vi "Drum Subvi.vi"(0 "Yellow Line":T2={"Global Rectangle"=[342, 292, 349, 377], "Contours"=[{"ID"=enum."External", "Type"=2, "Coordinates"=[342, 376, 348, 292]}]} {"Contours"."Type" items=["No Selection", "Point", "Line", "Rectangle", "Oval", "Polygon", "Freehand Region", "Annulus", "Unused2", "Unused3", "Broken Line", "Freehand Line", "Rotated Rectangle"]}, 1 "Green Line":T2={"Global Rectangle"=[406, 309, 423, 383], "Contours"=[{"ID"=enum."External", "Type"=2, "Coordinates"=[422, 382, 406, 309]}]} {"Contours"."Type" items=["No Selection", "Point", "Line", "Rectangle", "Oval", "Polygon", "Freehand Region", "Annulus", "Unused2", "Unused3", "Broken Line", "Freehand Line", "Rotated Rectangle"]}, 3 "Red Line":T2={"Global Rectangle"=[300, 297, 320, 380], "Contours"=[{"ID"=enum."External", "Type"=2, "Coordinates"=[300, 379, 319, 297]}]} {"Contours"."Type" items=["No Selection", "Point", "Line", "Rectangle", "Oval", "Polygon", "Freehand Region", "Annulus", "Unused2", "Unused3", "Broken Line", "Freehand Line", "Rotated Rectangle"]}, 8 "Image Dst Out":T1, 12 "Blue Line":T2={"Global Rectangle"=[374, 278, 383, 377], "Contours"=[{"ID"=enum."External", "Type"=2, "Coordinates"=[382, 376, 374, 278]}]} {"Contours"."Type" items=["No Selection", "Point", "Line", "Rectangle", "Oval", "Polygon", "Freehand Region", "Annulus", "Unused2", "Unused3", "Broken Line", "Freehand Line", "Rotated Rectangle"]}, 14 "error out":errorcluster) -> (7 "LED Red":bool, 9 "Yellow Array":bool[](array[boolean]), 13 "Foot Pedal":bool, 16 "Blue array":bool[](array[boolean]), 17 "Red Array":bool[](array[boolean]), 20 "Green Array":bool[](array[boolean]), 23 "Blue Drum 2":bool, 24 "Yellow Drum":bool, 25 "Green Drum":bool, 27 "error out 2":errorcluster)   [LabVIEW 2009]
uses:
  <vilib>/vision/Image Controls.llb/IMAQ Image.ctl
  <vilib>/Analysis/3filter.llb/Filter Passband Type.ctl
  <vilib>/Analysis/3filter.llb/Butterworth Filter (DBL).vi
  <vilib>/Analysis/NI_AALBase.lvlib
  <vilib>/vision/NI_Vision_Development_Module.lvlib
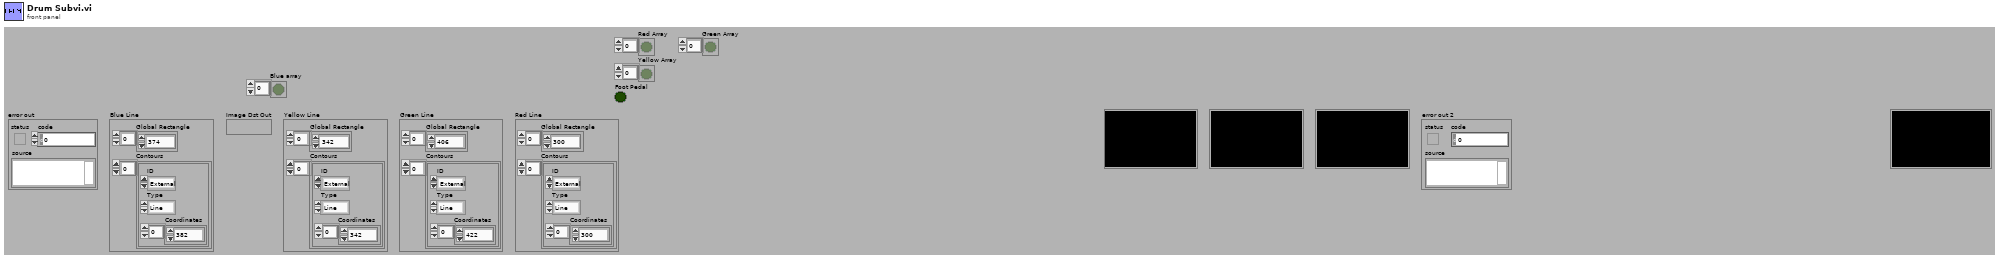
[diagram p1: front panel]
types:
  T1 = typedef "IMAQ Image.ctl" = refnum<image>
  T2 = cluster{"Global Rectangle":i32[], "Contours":cluster{"ID":enum32{"External", "Internal"}, "Type":u32, "Coordinates":i32[]}[]}
  T3 = typedef "NI_AALBase.lvlib/Filter Passband Type.ctl" = enum32{"Lowpass", "Highpass", "Bandpass", "Bandstop"}
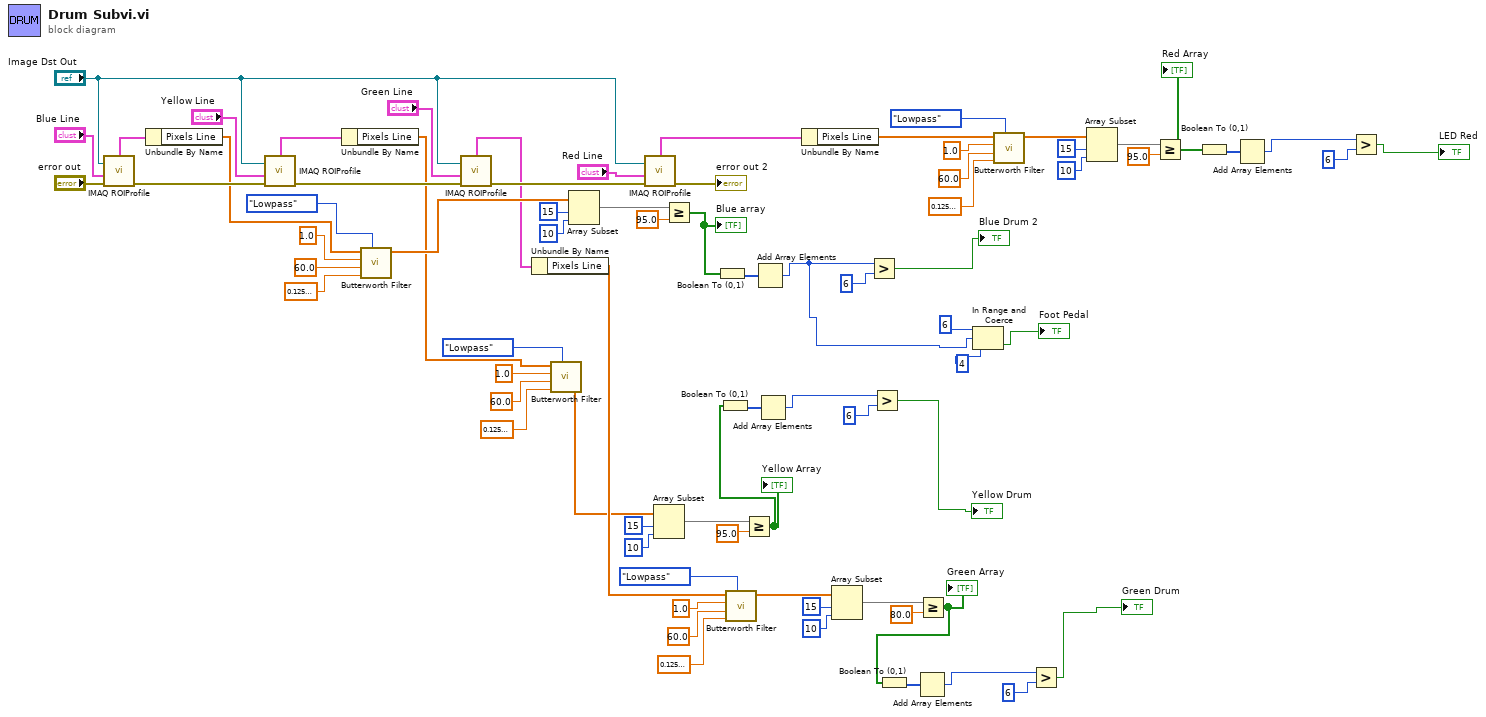
[diagram p0: block diagram]
diagram:
  n1 = call "IMAQ ROIProfile"("error in (no error)"="error out", "ROI Descriptor"="Blue Line", "Image"="Image Dst Out") -> ("error out"=w45:errorcluster, "ROI Graph"=w46:cluster{"x0":sgl, "dx":sgl, "Pixels Line":sgl[]})  [unwired: 4 out]
  n2 = Unbundle By Name(w46) -> ("Pixels Line"=w27:sgl[])
  n3 = call "IMAQ ROIProfile"("error in (no error)"=w45, "ROI Descriptor"="Yellow Line", "Image"="Image Dst Out") -> ("error out"=w74:errorcluster, "ROI Graph"=w42:cluster{"x0":sgl, "dx":sgl, "Pixels Line":sgl[]})  [unwired: 4 out]
  n4 = Unbundle By Name(w42) -> ("Pixels Line"=w39:sgl[])
  n5 = call-poly <vilib>:"Butterworth Filter.vi"("filter type"=Filter_Passband_Type."Lowpass", "low cutoff freq: fl"=0.12500000000000006 ("low"), "high cutoff freq: fh"=60.0 ("high"), "sampling freq: fs"=1.0 ("sampling"), "X"=w27) -> ("Filtered X"=w58:dbl[])  [unwired: 3 in, 1 out]
  n6 = call "IMAQ ROIProfile"("error in (no error)"=w74, "ROI Descriptor"="Green Line", "Image"="Image Dst Out") -> ("error out"=w71:errorcluster, "ROI Graph"=w48:cluster{"x0":sgl, "dx":sgl, "Pixels Line":sgl[]})  [unwired: 4 out]
  n7 = Unbundle By Name(w48) -> ("Pixels Line"=w51:sgl[])
  n8 = call-poly <vilib>:"Butterworth Filter.vi"("filter type"=Filter_Passband_Type."Lowpass", "low cutoff freq: fl"=0.12500000000000006 ("low  2"), "high cutoff freq: fh"=60.0 ("high 2"), "sampling freq: fs"=1.0 ("sampling 2"), "X"=w39) -> ("Filtered X"=w43:dbl[])  [unwired: 3 in, 1 out]
  n9 = Array Subset(array=w58, index=15, length=10) -> (w33:dbl[])
  n10 = call "IMAQ ROIProfile"("error in (no error)"=w71, "ROI Descriptor"="Red Line", "Image"="Image Dst Out") -> ("error out"=→"error out 2":errorcluster, "ROI Graph"=w69:cluster{"x0":sgl, "dx":sgl, "Pixels Line":sgl[]})  [unwired: 4 out]
  n11 = Array Subset(array=w43, index=15, length=10) -> (w36:dbl[])
  n12 = Greater Or Equal?(x=w33, y=95.0) -> (x >= y?=w21:bool[])
  "Blue array" <- w21
  n13 = Boolean To (0,1)(Boolean=w21) -> (0, 1=w20:i16[])
  n14 = call-poly <vilib>:"Butterworth Filter.vi"("filter type"=Filter_Passband_Type."Lowpass", "low cutoff freq: fl"=0.12500000000000006 ("low  3"), "high cutoff freq: fh"=60.0 ("high 3"), "sampling freq: fs"=1.0 ("sampling 3"), "X"=w51) -> ("Filtered X"=w47:dbl[])  [unwired: 3 in, 1 out]
  n15 = Greater Or Equal?(x=w36, y=95.0) -> (x >= y?=w7:bool[])
  "Yellow Array" <- w7
  n16 = Boolean To (0,1)(Boolean=w7) -> (0, 1=w14:i16[])
  n17 = Add Array Elements(numeric array=w20) -> (sum=w4:i16)
  n18 = Add Array Elements(numeric array=w14) -> (sum=w13:i16)
  n19 = Unbundle By Name(w69) -> ("Pixels Line"=w66:sgl[])
  n20 = Array Subset(array=w47, index=15, length=10) -> (w54:dbl[])
  n21 = Greater?(x=w4, y=6) -> (0:→"Blue Drum 2":bool)
  n22 = Greater?(x=w13, y=6) -> (0:→"Yellow Drum":bool)
  n23 = Greater Or Equal?(x=w54, y=80.0) -> (x >= y?=w8:bool[])
  "Green Array" <- w8
  n24 = Boolean To (0,1)(Boolean=w8) -> (0, 1=w11:i16[])
  n25 = Add Array Elements(numeric array=w11) -> (sum=w10:i16)
  n26 = In Range and Coerce(upper limit=6, x=w4, lower limit=4) -> (In Range?=→"Foot Pedal":bool)  [unwired: 1 out]
  n27 = call-poly <vilib>:"Butterworth Filter.vi"("filter type"=Filter_Passband_Type."Lowpass", "low cutoff freq: fl"=0.12500000000000006 ("low  4"), "high cutoff freq: fh"=60.0 ("high 4"), "sampling freq: fs"=1.0 ("sampling 4"), "X"=w66) -> ("Filtered X"=w70:dbl[])  [unwired: 3 in, 1 out]
  n28 = Greater?(x=w10, y=6) -> (0:→"Green Drum":bool)
  n29 = Array Subset(array=w70, index=15, length=10) -> (w63:dbl[])
  n30 = Greater Or Equal?(x=w63, y=95.0) -> (x >= y?=w17:bool[])
  "Red Array" <- w17
  n31 = Boolean To (0,1)(Boolean=w17) -> (0, 1=w18:i16[])
  n32 = Add Array Elements(numeric array=w18) -> (sum=w5:i16)
  n33 = Greater?(x=w5, y=6) -> (0:→"LED Red":bool)
